vi "Add File.vi"(8 "error in":errorcluster, 9 "Path":path, 10 "Project:Active Project":refnum<vi>) -> (0 "error out":errorcluster)   [LabVIEW 2021, in "_Rename.lvlib" / "_Rename.lvclass"]
uses:
  _Rename.lvclass
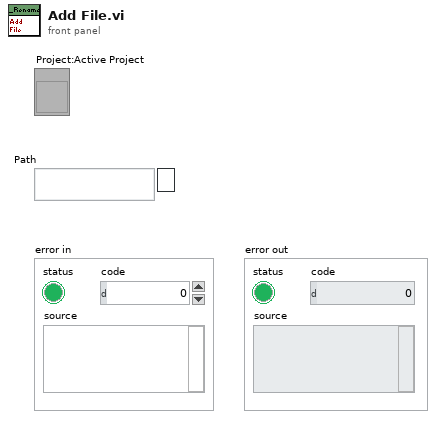
[diagram p1: front panel]
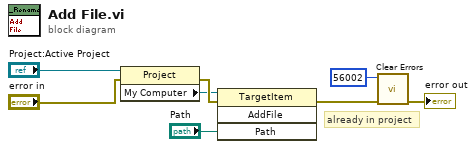
[diagram p0: block diagram]
diagram:
  # "already in project"
  n1 = property class="Project"(reference="Project:Active Project", error in="error in") -> (error out=w8:errorcluster, "My Computer"=w5:refnum<vi>)  [unwired: 1 out]
  n2 = invoke class="TargetItem" method="AddFile"(reference=w5, error in=w8, "Path"="Path") -> (error out=w7:errorcluster)  [unwired: 1 in, 3 out]
  n3 = call <vilib>:"Clear Errors.vi"("error in (no error)"=w7, "specific error code to clear (0: all)"=56002) -> ("error out"=→"error out":errorcluster)  [unwired: 4 in, 1 out]
